vi "feedback-boway.vi"(8 "error in (no error)":errorcluster, 10 "Move":T3, 11 "KNR in":T1) -> (0 "error out":errorcluster, 2 "Alpha":dbl, 3 "KNR out":T1)   [LabVIEW 2013]
uses:
  <userlib>/KNR OS 3.0 LabVIEW Toolkit/Type Definition/KNR3 Reference.ctl
  <userlib>/_FPGA Interface Advanced Tools/FPGA Interface Base/FPGA Interface Base.lvclass
  <userlib>/KNR OS 3.0 LabVIEW Toolkit/Type Definition/Resource.ctl
  <vilib>/Platform/TimedLoop/XDataNode/timing_clust.ctl
  <vilib>/Platform/TimedLoop/XDataNode/nitl_modes.ctl
  <vilib>/Platform/TimedLoop/XDataNode/wakeup.ctl
  Global_KNRm.vi
  <vilib>/platform/TimedLoop/XDataNode/XDataNode.xnode
  <vilib>/Platform/TimedLoop/XDataNode/XDNodeRunTimeDep.lvlib
panel:
  out "Time(sec)":dbl
  out "dirN":i32[](array[numeric])
  out "Pcmd 2":dbl
  out "Waveform Graph":dbl[][](graph)
  out "position":dbl[][](graph)
  out "PWM":dbl[][](graph)
  out "e":dbl
  out "dirPerr":dbl
  out "Boolean":bool
  out "Numeric":u32
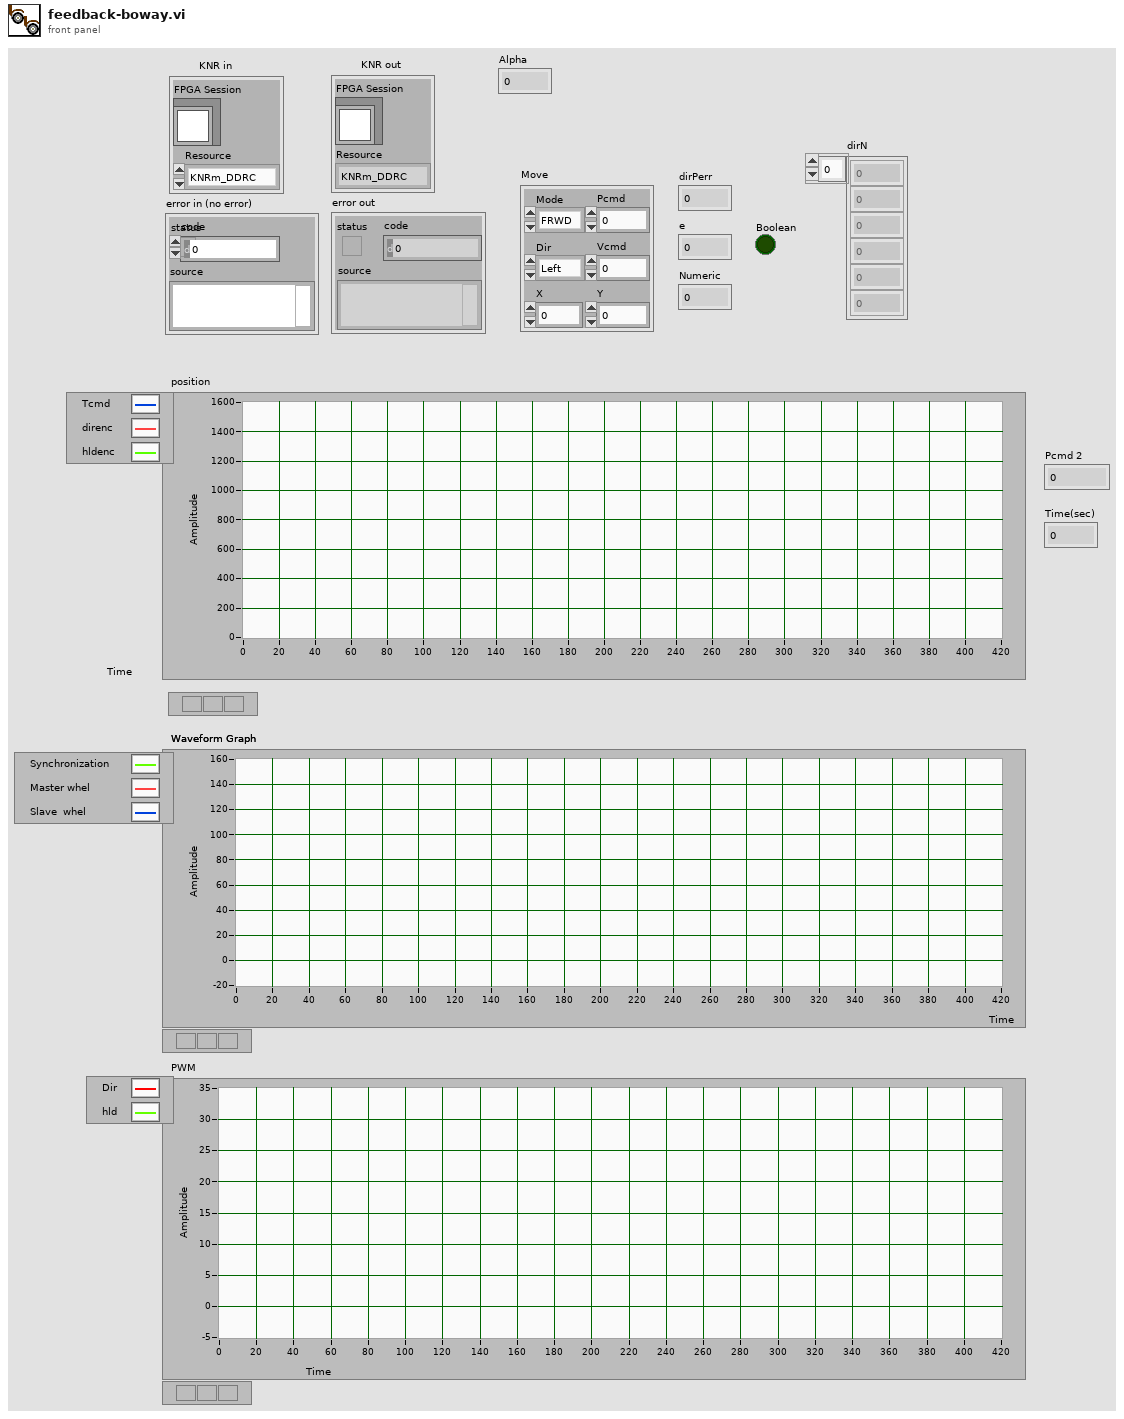
[diagram p1: front panel]
types:
  T1 = typedef "KNR3 Reference.ctl" = cluster{"FPGA Session":refnum<class "FPGA Interface Base.lvclass">, "Resource":T2}
  T2 = typedef "Resource.ctl" = enum16{"KNRm_DDRC", "KNRm_DDDD", "KNRm_DDDR", "KNRm_DDDC", "KNR"}
  T3 = cluster{"Mode":enum16{"FRWD", "TURFIX", "TURNOF", "CIRCULAR"}, "Dir":enum16{"Left", "Right"}, "Pcmd":dbl, "Vcmd":dbl, "X":dbl, "Y":dbl}
  T4 = cluster{"Nacc":i32, "deg":dbl, "cnt":i32, "Tacc":dbl, "Lest":dbl, "Ocmd":dbl, "Nc":i32, "Lmin":dbl, "Tcmd":dbl, "Tc":dbl, "Type":i32, "itrflg":i32}
  T5 = typedef "XDNodeRunTimeDep.lvlib/timing_clust.ctl" = cluster{"Expected End [f-1]":u64, "Actual End [f-1]":u64, "Finished Late? [f-1]":bool, "Expected End [i-1]":u64, "Actual End [i-1]":u64, "Finished Late? [i-1]":bool, "Expected Start [i]":u64, "Actual Start [i]":u64, "Expected Start [f]":u64, "Actual Start [f]":u64, "Source Name":string, "Structure Name":string, "Period":i64, "Deadline":i64, "Offset":i64, "Start":i64, "Priority":i32, "Timeout":i32, "Mode":T6, "Wakeup Reason":T7, "Error":errorcluster, "Source Type":string, "Secondary Source Type":string, "Global End Time":u64, "Global Start Time":u64, "Frame Duration":u64, "Iteration Duration":u64, "Assigned CPU":i32, "I/O Scan Engine Mode":u32}
  T6 = typedef "XDNodeRunTimeDep.lvlib/nitl_modes.ctl" = enum32{"No Change", "Process missed periods, maintain original phase", "Discard missed periods, maintain original phase", "Process missed periods, ignore original phase", "Discard missed periods, ignore original phase"}
  T7 = typedef "XDNodeRunTimeDep.lvlib/wakeup.ctl" = enum32{"Normal", "Aborted", "Asynchronous wakeup", "Timing source error", "Timed loop error", "Timeout"}
  T8 = cluster{"dir":cluster{"direnc":dbl, "direnc_b":dbl, "dirVerr_b":dbl, "dirU_b":dbl}, "hld":cluster{"hldenc":dbl, "hldenc_b":dbl, "hldVerr_b":dbl, "hldU_b":dbl}, "sc":cluster{"ei":dbl, "ed":dbl}}
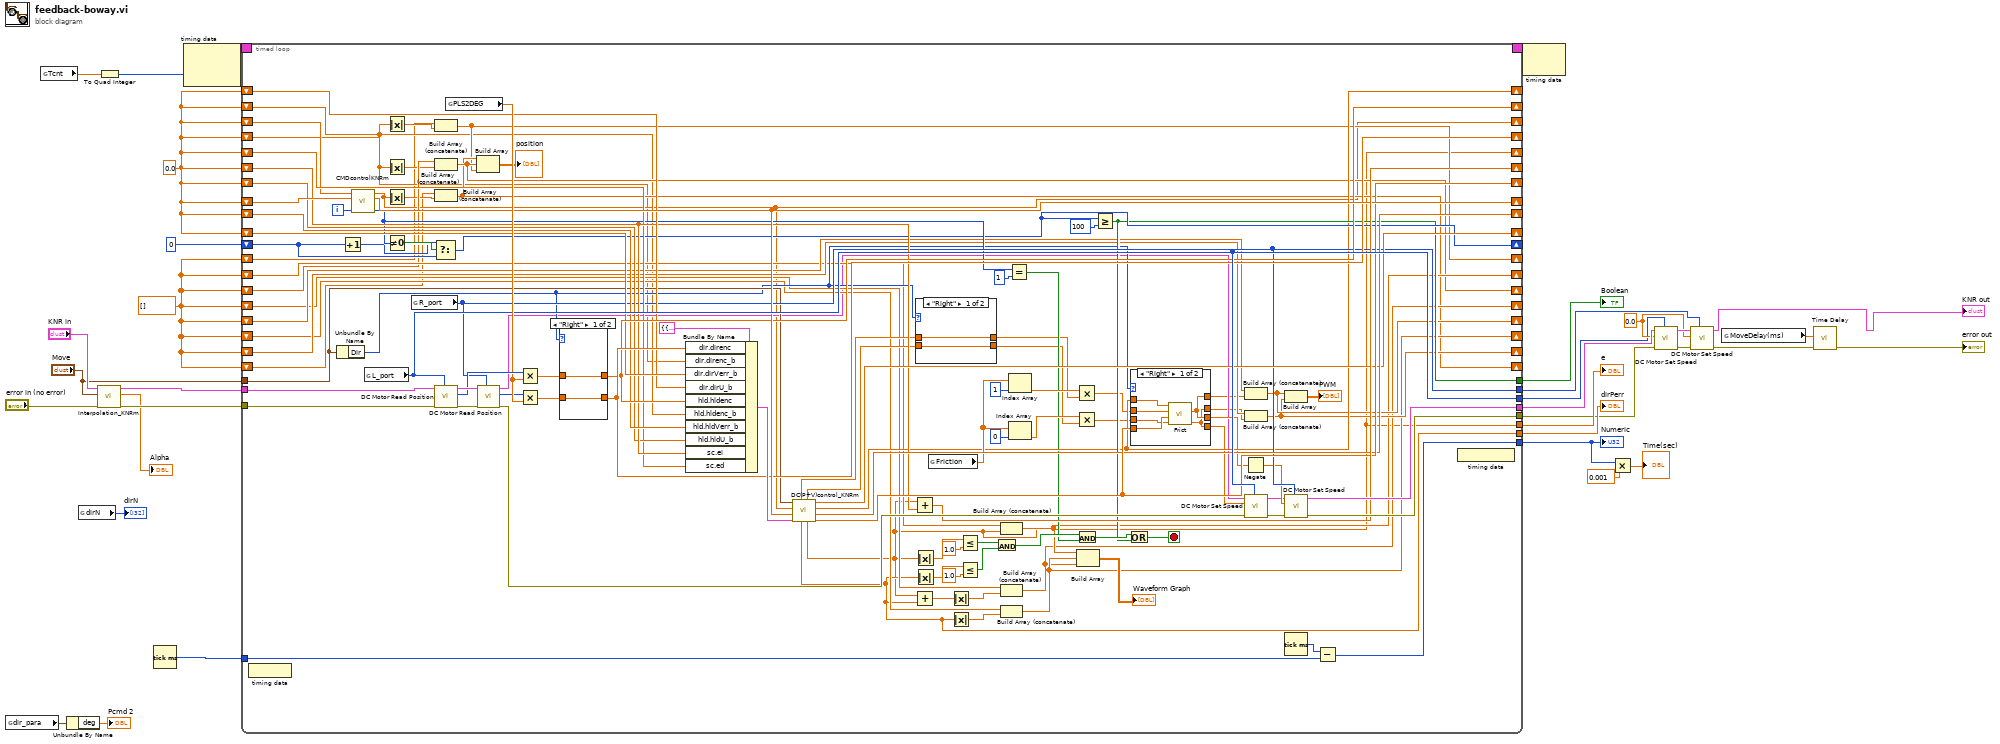
[diagram p0: block diagram]
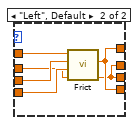
[diagram p3: hidden frame]
diagram:
  w14 = dbl[] []
  w24 = 0.0 ("hldVerr")
  w28 = 0.0 ("Speed (+-100%)")
  n1 = global read "Global_KNRm.vi" "dir_para"() -> (w10:T4)
  n2 = global read "Global_KNRm.vi" "Tcnt"() -> (w32:dbl)
  n3 = Unbundle By Name(w10) -> ("deg"=→"Pcmd 2":dbl)
  n4 = global read "Global_KNRm.vi" "dirN"() -> (→"dirN":i32[])
  n5 = call "Interpolation_KNRm.vi"("error in (no error)"="error in (no error)", "Move"="Move", "KNR in"="KNR in") -> ("error out"=w22:errorcluster, "Alpha"=→"Alpha":dbl, "KNR out"=w11:T1)  [unwired: 6 in]
  n6 = To Quad Integer(1:w32) -> (0:w31:i64)
  n7 = Tick Count (ms)() -> (millisecond timer value=w18:u32)
  n8 = node-c288(w31) -> (w34:T5)  [unwired: 1 in]
  n9 = timed-loop {
    timing: w34 -> [_]
    timing-out: [_] -> w33
    tunnel: "Move" -> [w83]
    tunnel: w11 -> [w138]
    tunnel: w22 -> [w137]
    tunnel: [w130] -> w30
    tunnel: [w129] -> w4
    tunnel: [w100] -> w26
    tunnel: [w128] -> w25
    shift-right: [w118] -> _
    shift-left: w24 -> [w103]
    shift-right: [w36] -> _
    shift-left: w24 -> [w101]
    shift-right: [w117] -> _
    shift-left: w24 -> [w111]
    shift-right: [w116] -> _
    shift-left: w24 -> [w102]
    shift-right: [w48] -> _
    shift-left: w24 -> [w42]
    shift-right: [w81] -> _
    shift-left: w24 -> [w104]
    shift-right: [w108] -> _
    shift-left: w24 -> [w37]
    shift-right: [w107] -> _
    shift-left: w24 -> [w50]
    shift-right: [w113] -> _
    shift-left: w24 -> [w105]
    shift-right: [w112] -> _
    shift-left: w24 -> [w106]
    shift-right: [w84] -> _
    shift-left: 0 -> [w95]
    tunnel: w18 -> [w92]
    tunnel: [w91] -> w3
    tunnel: [w82] -> w17
    tunnel: [w46] -> w16
    tunnel: [w36] -> w15
    shift-right: [w66] -> _
    shift-left: w14 -> [w65]
    shift-right: [w64] -> _
    shift-left: w14 -> [w63]
    shift-right: [w62] -> _
    shift-left: w14 -> [w61]
    shift-right: [w60] -> _
    shift-left: w14 -> [w59]
    shift-right: [w58] -> _
    shift-left: w14 -> [w57]
    shift-right: [w56] -> _
    shift-left: w14 -> [w52]
    shift-right: [w55] -> _
    shift-left: w14 -> [w38]
    shift-right: [w54] -> _
    shift-left: w14 -> [w35]
    i -> [w127]
    stop <- w97 stop-if-true
    n10 = node-c288() -> ()  [unwired: 1 in]
    n11 = Unbundle By Name(w83) -> ("Dir"=w78:enum16{"Left", "Right"})
    n12 = Increment(x=w95) -> (x+1=w94:i32)
    n13 = call "CMDcontrolKNRm.vi"("cnt"=w127, "prefed"=w111, "Tcmd"=w42) -> ("itrflg"=w99:i32, "Ocmd"=w117:dbl, "Tcmd"=w48:dbl)  [unwired: 6 in]
    n14 = global read "Global_KNRm.vi" "L_port"() -> (w128:i8)
    n15 = Absolute Value(x=w50) -> (abs(x)=w49:dbl)
    n16 = Absolute Value(x=w37) -> (abs(x)=w51:dbl)
    n17 = Absolute Value(x=w48) -> (abs(x)=w47:dbl)
    n18 = Not Equal To 0?(x=w99) -> (x != 0?=w96:bool)
    n19 = global read "Global_KNRm.vi" "R_port"() -> (w100:i8)
    n20 = Select(t=w94, s=w96, f=w95) -> (s? t:f=w84:i32)
    n21 = Build Array (concatenate)(w35, w49) -> (w54:dbl[])
    n22 = Build Array (concatenate)(w52, w51) -> (w56:dbl[])
    n23 = Build Array (concatenate)(w38, w47) -> (w55:dbl[])
    n24 = call <userlib>:"DC Motor Read Position.vi"("Port (DS1)"=w128, "error in (no error)"=w137, "KNR in"=w138) -> ("error out"=w136:errorcluster, "Position"=w135:i32, "KNR out"=w139:T1)  [unwired: 6 in]
    n25 = global read "Global_KNRm.vi" "PLS2DEG"() -> (w134:dbl)
    n26 = Build Array(w55, w56, w54) -> (→"position":dbl[][])
    n27 = call <userlib>:"DC Motor Read Position.vi"("Port (DS1)"=w100, "error in (no error)"=w136, "KNR in"=w139) -> ("error out"=w131:errorcluster, "Position"=w133:i32, "KNR out"=w53:T1)  [unwired: 6 in]
    n28 = Multiply(x=w135, y=w134) -> (x*y=w114:dbl)
    n29 = Multiply(x=w133, y=w134) -> (x*y=w115:dbl)
    n30 = case shown="\"Right\"" w78 {
      tunnel: [w156 w159] -> w108
      tunnel: w115 -> [w156 w158]
      tunnel: [w157 w158] -> w107
      tunnel: w114 -> [w157 w159]
      frame "Right" {
      }
      frame "Left", Default {
      }
    }
    n31 = Bundle By Name(cluster=T8 {"dir"={"direnc"=0.0, "direnc_b"=0.0, "dirVerr_b"=0.0, "dirU_b"=0.0}, "hld"={"hldenc"=0.0, "hldenc_b"=0.0, "hldVerr_b"=0.0, "hldU_b"=0.0}, "sc"={"ei"=0.0, "ed"=0.0}} ("control"), "dir.direnc"=w108, "dir.direnc_b"=w37, "dir.dirVerr_b"=w106, "dir.dirU_b"=w104, "hld.hldenc"=w107, "hld.hldenc_b"=w50, "hld.hldVerr_b"=w105, "hld.hldU_b"=w102, "sc.ei"=w103, "sc.ed"=w101) -> (w109:T8)
    n32 = call "DC(P+V)control_KNRm.vi"("control"=w109, "Ocmd"=w117, "Tcmd"=w48, "Move"=w83) -> ("hldU"=w116:dbl, "hldVerr"=w113:dbl, "dirU"=w81:dbl, "dirVerr"=w112:dbl, "e"=w36:dbl, "FriectH"=w76:dbl, "dirPerr"=w46:dbl, "FriectD"=w77:dbl)
    n33 = Add(x=w36, y=w103) -> (x+y=w118:dbl)
    n34 = Add(x=w36, y=w46) -> (x+y=w44:dbl)
    n35 = Absolute Value(x=w36) -> (abs(x)=w119:dbl)
    n36 = Absolute Value(x=w46) -> (abs(x)=w122:dbl)
    n37 = case shown="\"Right\"" w78 {
      tunnel: w77 -> [w141 w143]
      tunnel: [w140 w143] -> w73
      tunnel: w76 -> [w140 w142]
      tunnel: [w141 w142] -> w75
      frame "Right" {
      }
      frame "Left", Default {
      }
    }
    n38 = global read "Global_KNRm.vi" "Friction"() -> (w90:dbl[])
    n39 = Absolute Value(x=w44) -> (abs(x)=w43:dbl)
    n40 = Absolute Value(x=w46) -> (abs(x)=w45:dbl)
    n41 = Less Or Equal?(x=w119, y=1.0) -> (x <= y?=w121:bool)
    n42 = Less Or Equal?(x=w122, y=1.0) -> (x <= y?=w124:bool)
    n43 = And(x=w121, y=w124) -> (x .and. y?=w125:bool)
    n44 = Build Array (concatenate)(w61, w36) -> (w62:dbl[])
    n45 = Build Array (concatenate)(w57, w43) -> (w58:dbl[])
    n46 = Build Array (concatenate)(w59, w45) -> (w60:dbl[])
    n47 = Equal?(x=w99, y=1) -> (x = y?=w79:bool)
    n48 = Index Array(array=w90, index=1) -> (element=w86:dbl)
    n49 = Index Array(array=w90, index=0) -> (element=w87:dbl)
    n50 = Multiply(x=w86, y=w75) -> (x*y=w80:dbl)
    n51 = Multiply(x=w87, y=w73) -> (x*y=w74:dbl)
    n52 = And(x=w125, y=w79) -> (x .and. y?=w98:bool)
    n53 = Build Array(w62, w60, w58) -> (→"Waveform Graph":dbl[][])
    n54 = Greater Or Equal?(x=w84, y=100) -> (x >= y?=w82:bool)
    n55 = Or(x=w98, y=w82) -> (x .or. y?=w97:bool)
    n56 = case shown="\"Right\"" w78 {
      tunnel: w116 -> [w148 w154]
      tunnel: w81 -> [w149 w155]
      tunnel: [w145 w150] -> w69
      tunnel: [w144 w151] -> w72
      tunnel: w80 -> [w147 w152]
      tunnel: w74 -> [w146 w153]
      tunnel: [w145 w151] -> w40
      tunnel: [w144 w150] -> w41
      frame "Right" {
        n57 = call "Frict.vi"("FrictH"=w146, "hldU"=w148, "FrictD"=w147, "dirU"=w149) -> ("hldU"=w144:dbl, "dirU"=w145:dbl)  [unwired: 6 in]
      }
      frame "Left", Default {
        n58 = call "Frict.vi"("FrictH"=w152, "hldU"=w154, "FrictD"=w153, "dirU"=w155) -> ("hldU"=w150:dbl, "dirU"=w151:dbl)  [unwired: 6 in]
      }
    }
    n59 = Negate(x=w69) -> (-x=w70:dbl)
    n60 = Build Array (concatenate)(w65, w40) -> (w66:dbl[])
    n61 = Build Array (concatenate)(w63, w41) -> (w64:dbl[])
    n62 = call <userlib>:"DC Motor Set Speed.vi"("Port (DS1)"=w128, "error in (no error)"=w131, "Speed (+-100%)"=w72, "KNR in"=w53) -> ("error out"=w132:errorcluster, "KNR out"=w39:T1)  [unwired: 6 in]
    n63 = Build Array(w66, w64) -> (→"PWM":dbl[][])
    n64 = call <userlib>:"DC Motor Set Speed.vi"("Port (DS1)"=w100, "error in (no error)"=w132, "Speed (+-100%)"=w70, "KNR in"=w39) -> ("error out"=w129:errorcluster, "KNR out"=w130:T1)  [unwired: 6 in]
    n65 = Tick Count (ms)() -> (millisecond timer value=w93:u32)
    n66 = Subtract(x=w93, y=w92) -> (x-y=w91:u32)
    n67 = node-c288() -> ()  [unwired: 1 out]
  }
  "Numeric" <- w3
  "Boolean" <- w17
  "dirPerr" <- w16
  "e" <- w15
  n68 = node-c288(w33) -> ()  [unwired: 1 out]
  n69 = Multiply(x=w3, y=0.001) -> (x*y=→"Time(sec)":dbl)
  n70 = call <userlib>:"DC Motor Set Speed.vi"("Port (DS1)"=w25, "error in (no error)"=w4, "Speed (+-100%)"=w28, "KNR in"=w30) -> ("error out"=w27:errorcluster, "KNR out"=w29:T1)  [unwired: 6 in]
  n71 = call <userlib>:"DC Motor Set Speed.vi"("Port (DS1)"=w26, "error in (no error)"=w27, "Speed (+-100%)"=w28, "KNR in"=w29) -> ("error out"=w13:errorcluster, "KNR out"=→"KNR out":T1)  [unwired: 6 in]
  n72 = global read "Global_KNRm.vi" "MoveDelay(ms)"() -> (w19:dbl)
  n73 = call "Time Delay"("error in (no error)"=w13, "Delay Time (s)"=w19) -> ("error out"=→"error out":errorcluster)  [unwired: 9 in]
